vi "AutoBike FPGA backup.vi"() -> ()   [LabVIEW 2016]
doc: "The roboRIO FPGA Shipping Personality. This personality supports:\n- 8 Analog Input channels with 1 sample\n- 2 Analog Output channels with 1 sample\n- 30 Digital I/O channels with 1 sample\n- 1 RSL channel\n- 4 Relay channels\n- 1 Button\n- 3 LEDs\n- 1 Accelerometer\n- 13 PWM channels\n- 6 Encoder channels\n- 2 SPI channels\n- 2 I2C channels\n- 2 UART channels\n- 1 CAN channel\n- 2 Analog Input Interrupt\n- 5 Digital Input Interrupt\n- 1 Timer Interrupt"
uses:
  <vilib>/Platform/TimedLoop/XDataNode/wakeup.ctl
  <vilib>/Platform/TimedLoop/XDataNode/XDNodeRunTimeDep.lvlib
  <vilib>/Platform/TimedLoop/XDataNode/nitl_modes.ctl
  <vilib>/Platform/TimedLoop/XDataNode/timing_clust.ctl
  <vilib>/Platform/TimedLoop/XDataNode/XDataNode.xnode
  <vilib>/eio/EIONode/EIONode.xnode
  <vilib>/rvi/eio/common/nirviEmuTemplateMethod_errors.vi
  <vilib>/rvi/LocalResourceManager/LocalResourceManager.xnode
  <vilib>/rvi/DataTransferAndStorage/Container/Common/niFpgaContainerGetUniqueNameForEmu.vi
  <vilib>/rvi/DataTransferAndStorage/Container/Common/niFpgaContainerSetEmuInfo.vi
  <vilib>/rvi/eio/common/nirviEmuReportErrorAndStop.vi
  <vilib>/rvi/DataTransferAndStorage/Container/XNode/niFpgaContainer.xnode
  <vilib>/rvi/FIFO/Fifo_Resource/nirvififoEmulationRead.vi
  <vilib>/rvi/FIFO/Fifo_Resource/nirvififoEmulationWrite.vi
  Sub VIs/Utilities/Start Boolean.ctl
panel:
  out "DIO.SPI_CS3:0.IN":u8 format="%08b"
  in  "DIO.SPI_CS3:0.DIR":u8 format="%08b"
  in  "DIO.SPI_CS3:0.OUT":u8 format="%08b"
  in  "IRQ.TIMER.SETTIME":T1
  in  "IRQ.TIMER.WRITE":u32
  out "IRQ.TIMER.READ":u32
  in  "IRQ.DI_BTN.NO":u8
  in  "IRQ.DI_BTN.CNT":u32
  in  "IRQ.DI_BTN.FALL":bool
  in  "IRQ.DI_BTN.RISE":bool
  in  "IRQ.DI_BTN.ENA":bool
  in  "IRQ.AI_B_0.HYSTERESIS":u16=17
  in  "IRQ.AI_B_1.HYSTERESIS":u16=17
  in  "IRQ.AI_B_1.NO":u8
  in  "IRQ.AI_B_0.NO":u8
  in  "IRQ.AI_B_1.THRESHOLD":u16
  in  "IRQ.AI_B_0.THRESHOLD":u16
  in  "IRQ.AI_B_3:0.CNFG":u8 format="%.0b"
  in  "IRQ.DIO_B_0.NO":u8
  in  "IRQ.DIO_B_1.NO":u8
  in  "IRQ.DIO_B_2.NO":u8
  in  "IRQ.DIO_B_3.NO":u8
  in  "IRQ.DIO_B_3.CNT":u32
  in  "IRQ.DIO_B_2.CNT":u32
  in  "IRQ.DIO_B_1.CNT":u32
  in  "IRQ.DIO_B_0.CNT":u32
  in  "IRQ.DIO_B_7:0.FALL":u8 format="%08b"
  in  "IRQ.DIO_B_7:0.RISE":u8 format="%08b"
  in  "IRQ.DIO_B_7:0.ENA":u8 format="%08b"
  in  "SPI.SPI.IRQ.NO":u8=15
  in  "SPI.B.IRQ.NO":u8=15
  out "DIO.DIO_9:8.IN":u8 format="%08b"
  in  "ENC.DIO_3.CNFG":u8 format="%08b"
  out "ENC.DIO_3.CNTR":u32
  out "ENC.DIO_3.STAT":u8 format="%08b"
  in  "ENC.DIO_4.CNFG":u8 format="%08b"
  out "ENC.DIO_4.CNTR":u32
  out "ENC.DIO_4.STAT":u8 format="%08b"
  in  "DIO.DIO_9:8.OUT":u8 format="%08b"
  in  "DIO.DIO_9:8.DIR":u8 format="%08b"
  in  "ENC.DIO_2.CNFG":u8 format="%08b"
  out "ENC.DIO_2.CNTR":u32
  out "ENC.DIO_2.STAT":u8 format="%08b"
  out "ENC.DIO_1.STAT":u8 format="%08b"
  out "ENC.DIO_1.CNTR":u32
  in  "ENC.DIO_1.CNFG":u8 format="%08b"
  out "DIO.DIO_7:0.IN":u8 format="%08b"
  in  "SYS.SELECTDIO":u8 format="%08b"
  in  "DIO.DIO_7:0.DIR":u8 format="%08b"
  in  "DIO.DIO_7:0.OUT":u8 format="%08b"
  out "ENC.DIO_0.STAT":u8 format="%08b"
  out "ENC.DIO_0.CNTR":u32
  in  "ENC.DIO_0.CNFG":u8 format="%08b"
  out "DI.BTN":u8 format="%08b"
  in  "DO.LED 5:0":u8 format="%06b"
  in  "DO.RSL.OUT":bool
  out "SPI.SPI.STAT":u8 format="%08b"
  in  "SPI.SPI.GO":T1
  in  "SPI.SPI.CNT":u16
  in  "SPI.SPI.CNFG":u16 format="%016b"
  out "SPI.SPI.DATI":u16
  in  "SPI.SPI.DATO":u16
  out "I2C.I2C.DATI":u8
  out "I2C.I2C.STAT":u8 format="%08b"
  in  "I2C.I2C.DATO":u8
  in  "I2C.I2CADDR":u8 format="%08b"
  in  "I2C.I2C.CNTR":u8
  in  "I2C.I2C.CNTL":u8 format="%08b"
  in  "I2C.I2C.CNFG":u8 format="%08b"
  in  "I2C.I2C.GO":T1
  out "ACC.Z.VAL":u16
  out "ACC.Y.VAL":u16
  out "ACC.X.VAL":u16
  in  "DO.RELAY.OUT":u8 format="%08b"
  out "SYS.ACC.RDY":bool
  out "SYS.RDY":bool
  in  "PWM.PWM_5.MAX":u16
  in  "PWM.PWM_5.CMP":u16
  in  "PWM.PWM_5.CNFG":u8 format="%08b"
  in  "PWM.PWM_5.CS":u8
  out "PWM.PWM_5.CNTR":u16
  in  "PWM.PWM_6.MAX":u16
  in  "PWM.PWM_6.CMP":u16
  in  "PWM.PWM_6.CNFG":u8 format="%08b"
  in  "PWM.PWM_6.CS":u8
  out "PWM.PWM_6.CNTR":u16
  in  "PWM.PWM_7.MAX":u16
  in  "PWM.PWM_7.CMP":u16
  in  "PWM.PWM_7.CNFG":u8 format="%08b"
  in  "PWM.PWM_7.CS":u8
  out "PWM.PWM_7.CNTR":u16
  in  "PWM.PWM_8.MAX":u16
  in  "PWM.PWM_8.CMP":u16
  in  "PWM.PWM_8.CNFG":u8 format="%08b"
  in  "PWM.PWM_8.CS":u8
  out "PWM.PWM_8.CNTR":u16
  in  "PWM.PWM_9.MAX":u16
  in  "PWM.PWM_9.CMP":u16
  in  "PWM.PWM_9.CNFG":u8 format="%08b"
  in  "PWM.PWM_9.CS":u8
  out "PWM.PWM_9.CNTR":u16
  in  "PWM.PWM_4.MAX":u16
  in  "PWM.PWM_4.CMP":u16
  in  "PWM.PWM_4.CNFG":u8 format="%08b"
  in  "PWM.PWM_4.CS":u8
  out "PWM.PWM_4.CNTR":u16
  in  "PWM.PWM_3.MAX":u16
  in  "PWM.PWM_3.CMP":u16
  in  "PWM.PWM_3.CNFG":u8 format="%08b"
  in  "PWM.PWM_3.CS":u8
  out "PWM.PWM_3.CNTR":u16
  in  "PWM.PWM_2.MAX":u16
  in  "PWM.PWM_2.CMP":u16
  in  "PWM.PWM_2.CNFG":u8 format="%08b"
  in  "PWM.PWM_2.CS":u8
  out "PWM.PWM_2.CNTR":u16
  in  "PWM.PWM_1.MAX":u16
  in  "PWM.PWM_1.CMP":u16
  in  "PWM.PWM_1.CNFG":u8 format="%08b"
  in  "PWM.PWM_1.CS":u8
  out "PWM.PWM_1.CNTR":u16
  out "PWM.PWM_0.CNTR":u16
  in  "PWM.PWM_0.CS":u8
  in  "PWM.PWM_0.CNFG":u8 format="%08b"
  in  "PWM.PWM_0.CMP":u16
  in  "PWM.PWM_0.MAX":u16
  in  "AO.B_0.VAL":u16
  in  "AO.B_1.VAL":u16
  in  "AO.SYS.GO":T1
  out "AO.SYS.STAT":bool
  out "AI.B_0.VAL":u16
  out "AI.B_1.VAL":u16
  out "AI.B_2.VAL":u16
  out "AI.B_3.VAL":u16
  out "AI.AI_0.VAL":u16
  out "AI.AI_1.VAL":u16
  out "AI.AI_2.VAL":u16
  out "AI.AI_3.VAL":u16
  out "SYS.AI.RDY":bool
  in  "SYS.SELECTB":u8 format="%08b"
  in  "DIO.B_7:0.OUT":u8 format="%08b"
  in  "DIO.B_7:0.DIR":u8 format="%08b"
  out "DIO.B_7:0.IN":u8 format="%08b"
  in  "DIO.B_15:8.OUT":u8 format="%08b"
  in  "DIO.B_15:8.DIR":u8 format="%08b"
  out "DIO.B_15:8.IN":u8 format="%08b"
  in  "SPI.B.DATO":u16
  out "SPI.B.DATI":u16
  in  "SPI.B.CNFG":u16 format="%016b"
  in  "SPI.B.CNT":u16
  in  "SPI.B.GO":T1
  out "SPI.B.STAT":u8 format="%08b"
  in  "PWM.B_0.MAX":u16
  in  "PWM.B_0.CMP":u16
  in  "PWM.B_0.CNFG":u8 format="%08b"
  in  "PWM.B_0.CS":u8
  out "PWM.B_0.CNTR":u16
  in  "PWM.B_1.CMP":u16
  in  "PWM.B_1.MAX":u16
  out "PWM.B_1.CNTR":u16
  in  "PWM.B_1.CNFG":u8 format="%08b"
  in  "PWM.B_1.CS":u8
  in  "PWM.B_2.CMP":u16
  in  "PWM.B_2.MAX":u16
  out "PWM.B_2.CNTR":u16
  in  "PWM.B_2.CNFG":u8 format="%08b"
  in  "PWM.B_2.CS":u8
  in  "I2C.B.DATO":u8
  out "I2C.B.DATI":u8
  in  "I2C.B.ADDR":u8 format="%08b"
  in  "I2C.B.CNTR":u8
  in  "I2C.B.CNTL":u8 format="%08b"
  out "I2C.B.STAT":u8 format="%08b"
  in  "I2C.B.CNFG":u8 format="%08b"
  in  "I2C.B.GO":T1
  in  "ENC.B.CNFG":u8 format="%08b"
  out "ENC.B.CNTR":u32
  out "ENC.B.STAT":u8 format="%08b"
  # "System"
  # "Onboard Devices"
  # "Connector B"
  # "DIO"
  # "SPI"
  # "PWM"
  # "I2C"
  # "AI"
  # "RELAY"
  # "RSL"
  # "Accelerometer"
  # "SPI Master"
  # "Analog Input"
  # "Analog Output"
  # "Digital I/O"
  # "Counters / PWM"
  # "Digital I/O"
  # "Encoders"
  # "IO Configuration"
  # "Buttons & LEDs"
  # "SPI CS DIO"
  # "Analog Interrupt"
  # "Digital Interrupt"
  # "Encoders"
  # "IO Configuration"
  # "Button Interrupt"
  # "I2C Master"
  # "FPGA Timer"
  # "This VI contains the default FPGA personality in addition to code that generates a sine waveform and filtered sine waveform based on parameters set by RT Main.vi. Keeping the default personality allows you to continue using the roboRIO APIs even after adding custom FPGA code."
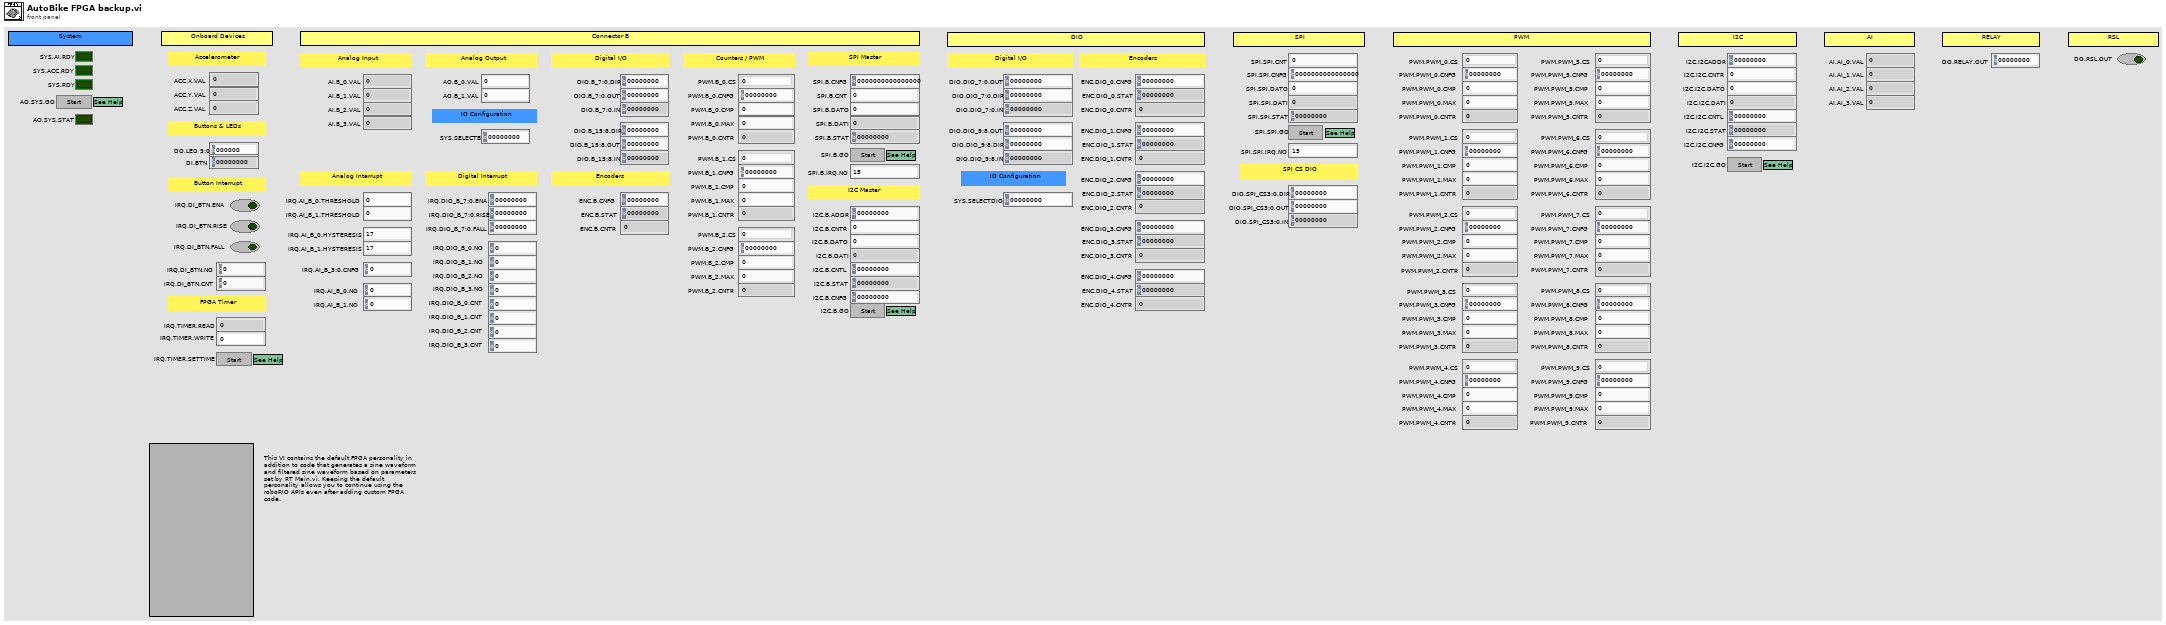
[diagram p1: front panel]
types:
  T1 = typedef "Start Boolean.ctl" = bool
  T2 = typedef "XDNodeRunTimeDep.lvlib/timing_clust.ctl" = cluster{"Expected End [f-1]":u64, "Actual End [f-1]":u64, "Finished Late? [f-1]":bool, "Expected End [i-1]":u64, "Actual End [i-1]":u64, "Finished Late? [i-1]":bool, "Expected Start [i]":u64, "Actual Start [i]":u64, "Expected Start [f]":u64, "Actual Start [f]":u64, "Source Name":string, "Structure Name":string, "Period":i64, "Deadline":i64, "Offset":i64, "Start":i64, "Priority":i32, "Timeout":i32, "Mode":T3, "Wakeup Reason":T4, "Error":errorcluster, "Source Type":string, "Secondary Source Type":string, "Global End Time":u64, "Global Start Time":u64, "Frame Duration":u64, "Iteration Duration":u64, "Assigned CPU":i32, "I/O Scan Engine Mode":u32}
  T3 = typedef "XDNodeRunTimeDep.lvlib/nitl_modes.ctl" = enum32{"No Change", "Process missed periods, maintain original phase", "Discard missed periods, maintain original phase", "Process missed periods, ignore original phase", "Discard missed periods, ignore original phase"}
  T4 = typedef "XDNodeRunTimeDep.lvlib/wakeup.ctl" = enum32{"Normal", "Aborted", "Asynchronous wakeup", "Timing source error", "Timed loop error", "Timeout"}
diagram:
  # "The accelerometer nodes take some time before the FPGA can first read the values. This is because it takes time to read from the accelerometer. An iteration of the While Loop will not complete until the accelerometer values have been read.\n\nAfter the completion of the first iteration of the While Loop, all indicators have valid values."
  # "The analog output nodes take some time before the FPGA write the values to the pins. The GO and STAT registers are used to handshake between the FPGA and host. When the host wants the values to be written, the host sets the GO register to TRUE. If the host reads the STAT register before setting the value of the GO register, it can wait for the value of the STAT register to invert. The value inversion tells the host that the output values have been written."
  # "The FPGA timer fires the interrupt request (IRQ) when TIMER.Read counts down to zero. If TIMER.Read is not zero, it counts down to one per microsecond."
  # "The analog input nodes take some time before the FPGA can first read the values. This is because it takes time to set up the Analog-to-Digital converter (ADC) and convert the first reading. An iteration of the While Loop will not complete until all the analog input channels have been sampled.\n\nAfter the completion of the first iteration of the While Loop, all indicators have valid values."
  # "Note: On some hardware a \"ghosting effect\" may occur on any unconnected AI channels. For example, if channel AI0 is connected and channels AI1~AI7 are not connected the the value read at AI0 may be seen on indicators AI1~AI7. This is common for hardware that use a multiplexed (MUXed) Analog-to-Digital converter (ADC), because the input analog signal is used to charge a capacitor which does not discharge before the unconnected channel is read.\n\nYou can hide the \"ghosting effect\" by using an mask register. This register is used to decide when the indicator should be updated."
  # "The only interface that sends interrupts to the RT side. Timer interrupts, analog input interrupts, digital input interrupts, and SPI interrupt share this interface.\n\nAll interrupts work in sequence. One interrupt waits until the previous interrupt request (IRQ) gets acknowledged on the RT side."
  # "NOTE: The SYS.RDY boolean MUST exist and must become TRUE at some point otherwise the myRIO API will not function correctly."
  # "There is some delay between when the FPGA code starts and the analog inputs, accelerometer, and scaling values outputs are valid. If the host wants to ensure that there are valid values in theses registers it should wait for each subsystem to finish its initialization process. \n\nWhen all subsystems have finished initializinig, the SYS.RDY indicator will be true, which can be polled by the host to determine the status of the FPGA. Alternatively, the host can poll the individual SYS.xx.RDY indicators to determine the status of the individual subsystems.\n\nThis loop continues indefinitely, essentially making SYS.RDY a read-only register."
  n1 = while {
    stop <- FALSE stop-if-true
    # "Host Synchronization"
    n2 = local read "SYS.ACC.RDY"() -> (w23:bool)
    n3 = local read "SYS.AI.RDY"() -> (w25:bool)
    n4 = Compound Arithmetic op=AND(w25, w23) -> (→"SYS.RDY":bool)
  }
  n5 = while {
    stop <- FALSE stop-if-true
    # "Interrupt to RT"
    n6 = xnode ("FIFO Method Node")("Timeout"=-1) -> ("Element"=w28:u8)  [unwired: 1 in, 2 out]
    n7 = call <vilib>:"niFPGA Interrupt.vi"("Wait Until Cleared (F)"=TRUE, "IRQ Number (0)"=w28) -> ()  [unwired: 1 in]
  }
  n8 = while {
    stop <- FALSE stop-if-true
    # "Timer"
    n9 = local read "IRQ.TIMER.READ"() -> (w33:u32)
    n10 = Select(t="IRQ.TIMER.WRITE", s="IRQ.TIMER.SETTIME", f=w33) -> (s? t:f=w31:u32)
    n11 = case shown="Default" w31 {
      selector: w31 -> [w37 w40]
      tunnel: [w37 w38] -> w30
      frame 0 {
      }
      frame Default {
        n12 = Decrement(x=w40) -> (x-1=w39:u32)
        n13 = case shown="0" w39 {
          selector: w39 -> [w41 w44]
          tunnel: [w41 w44] -> w38
          frame Default {
          }
          frame 0 {
            w43 = u8 0  # Reserved for Timer IRQ
            n14 = xnode ("FIFO Method Node")("Element"=w43, "Timeout"=-1) -> ()  [unwired: 1 in, 2 out]
          }
        }
      }
    }
    "IRQ.TIMER.READ" <- w30
    n15 = call "Loop Timer"("Count(uSec)"=u8 1 ("Count(mSec)")) -> ()  [unwired: 1 out]
  }
  n16 = xnode "VI-Defined FIFO Configuration"() -> ("FIFO Out"=w2:refnum<k21>)
  n17 = while {
    tunnel: w2 -> [w53]
    i -> [w67]
    stop <- FALSE stop-if-true
    # "Analog Input"
    n18 = Greater Than 0?(x=w67) -> (x > 0?=→"SYS.AI.RDY":bool)
    n19 = xnode "FPGA I/O Node"() -> ("MXP/AI0"=w46, "MXP/AI1"=w45, "MXP/AI2"=→"AI.B_2.VAL", "MXP/AI3"=→"AI.B_3.VAL", "AnalogIn0"=→"AI.AI_0.VAL", "AnalogIn1"=→"AI.AI_1.VAL", "AnalogIn2"=→"AI.AI_2.VAL", "AnalogIn3"=→"AI.AI_3.VAL")  [unwired: 8 in, 8 out]
    "AI.B_0.VAL" <- w46
    "AI.B_1.VAL" <- w45
    n20 = Number To Boolean Array(number="IRQ.AI_B_3:0.CNFG") -> (Boolean array=w54:bool[])
    n21 = Index Array(array=w54) -> (element #1=w56:bool, element #2=w57:bool, element #3=w59:bool, element #4=w60:bool)  [unwired: 4 in]
    n22 = call "Check AI IRQ.vi"("Hysteresis"="IRQ.AI_B_1.HYSTERESIS", "FIFO In"=w53, "IRQ Number"="IRQ.AI_B_1.NO", "Threshold"="IRQ.AI_B_1.THRESHOLD", "Analog Value"=w45, "Rising Edge?"=w60, "Enable Interrupt?"=w59) -> ()  [unwired: 5 in]
    n23 = call "Check AI IRQ.vi"("Hysteresis"="IRQ.AI_B_0.HYSTERESIS", "FIFO In"=w53, "IRQ Number"="IRQ.AI_B_0.NO", "Threshold"="IRQ.AI_B_0.THRESHOLD", "Analog Value"=w46, "Rising Edge?"=w57, "Enable Interrupt?"=w56) -> ()  [unwired: 5 in]
  }
  n24 = while {
    stop <- FALSE stop-if-true
    # "Analog Output"
    n25 = feedback #1(FALSE) -> (w71:bool)
    n26 = case shown="True" "AO.SYS.GO" {
      tunnel: "AO.B_0.VAL" -> [_ w81]
      tunnel: "AO.B_1.VAL" -> [_ w80]
      tunnel: w71 -> [w76 w79]
      tunnel: [w76 w77] -> w69
      frame False {
      }
      frame True {
        n27 = flat-sequence {
          tunnel: w81 -> [w84]
          tunnel: w80 -> [w83]
          tunnel: w79 -> [w82]
          tunnel: [w82] -> w78
          tunnel: w78 -> [w86]
          tunnel: [w85] -> w77
          frame #0 {
            n28 = xnode "FPGA I/O Node"("MXP/AO0"=w84, "MXP/AO1"=w83) -> ()  [unwired: 2 in, 2 out]
          }
          frame #1 {
            n29 = Not(x=w86) -> (.not. x?=w85:bool)
          }
        }
      }
    }
    "AO.SYS.STAT" <- w69
    n30 = feedback-in #1(w69) -> ()
  }
  n31 = while {
    i -> [w94]
    stop <- FALSE stop-if-true
    # "Onboard Accelerometer"
    n32 = xnode "FPGA I/O Node"() -> ("AccelerationX"=w92, "AccelerationY"=w91, "AccelerationZ"=w90)  [unwired: 3 in, 3 out]
    n33 = Greater Than 0?(x=w94) -> (x > 0?=→"SYS.ACC.RDY":bool)
    n34 = To Unsigned Word Integer(number=w92) -> (unsigned 16bit integer=→"ACC.X.VAL":u16)
    n35 = To Unsigned Word Integer(number=w91) -> (unsigned 16bit integer=→"ACC.Y.VAL":u16)
    n36 = To Unsigned Word Integer(number=w90) -> (unsigned 16bit integer=→"ACC.Z.VAL":u16)
  }
  n37 = xnode "VI-Defined FIFO Configuration"() -> ("FIFO Out"=w1:refnum<k21>)
  n38 = node-c288() -> (w7:T2)  [unwired: 1 in]
  n39 = timed-loop {
    timing: w7 -> [_]
    timing-out: [_] -> w6
    tunnel: w1 -> [w101]
    stop <- FALSE stop-if-true
    # "Button IRQ"
    # "Onboard DIO"
    n40 = xnode "FPGA I/O Node"() -> ("User Button"=w102)  [unwired: 1 in, 1 out]
    n41 = Number To Boolean Array(number="DO.LED 5:0") -> (Boolean array=w112:bool[])
    n42 = Index Array(array=w112) -> (element #1=w110:bool, element #2=w109:bool, element #3=w108:bool, element #4=w107:bool, element #5=w106:bool, element #6=w105:bool)  [unwired: 6 in]
    n43 = Build Array(w102) -> (w104:void[])
    n44 = call "DIO IRQ 1-bit.vi"("IRQ.NO"="IRQ.DI_BTN.NO", "IRQ.CNT"="IRQ.DI_BTN.CNT", "FIFO in"=w101, "IRQ.FALL"="IRQ.DI_BTN.FALL", "IRQ.RISE"="IRQ.DI_BTN.RISE", "IRQ.ENA"="IRQ.DI_BTN.ENA", "DIO"=w102) -> ()  [unwired: 5 in]
    n45 = Boolean Array To Number(Boolean array=w104) -> (number=→"DI.BTN":u8)
    n46 = xnode "FPGA I/O Node"("Radio LED Green"=w110, "Radio LED Red"=w109, "Comm LED Green"=w108, "Comm LED Red"=w107, "Mode LED Green"=w106, "Mode LED Red"=w105) -> ()  [unwired: 6 in, 6 out]
  }
  n47 = while {
    stop <- FALSE stop-if-true
    # "Button SCTL Interrupt Buffer"
    n48 = feedback #2(u8 0 ("Element")) -> (w118:u8)
    n49 = feedback #3(FALSE ("Timed Out?")) -> (w122:bool)
    n50 = case shown="False" w122 {
      tunnel: [w124 w126] -> w119
      tunnel: w118 -> [_ w126]
      frame False {
        n51 = xnode ("FIFO Read")("Timeout"=-1) -> ("Element"=w124:u8)  [unwired: 1 in, 2 out]
      }
      frame True {
      }
    }
    n52 = feedback-in #2(w119) -> ()
    n53 = xnode ("FIFO Method Node")("Element"=w119, "Timeout"=0) -> ("Timed Out?"=w120:bool)  [unwired: 1 in, 1 out]
    n54 = feedback-in #3(w120) -> ()
  }
  n55 = node-c288(w6) -> ()
  n56 = xnode "VI-Defined FIFO Configuration"() -> ("FIFO Out"=w5:refnum<k21>)
  n57 = xnode "VI-Defined FIFO Configuration"() -> ("FIFO Out"=w3:refnum<k21>)
  n58 = node-c288() -> (w21:T2)  [unwired: 1 in]
  n59 = timed-loop {
    timing: w21 -> [_]
    timing-out: [_] -> w20
    tunnel: w5 -> [w163]
    tunnel: w3 -> [w151]
    stop <- _ stop-if-true
    # "DIO/ IRQ"
    # "DIO / Encoder"
    # "DIO / I2C Master"
    # "DIO / PWM"
    # "DIO"
    # "DIO"
    # "DIO/ SPI Master"
    # "Connector MXP DIO"
    n60 = call "Split HDC Bank1 DIO.vi"("IN 7:0"="DIO.B_7:0.OUT") -> ("OUT 3:0"=w251:fxp<+,4,4>, "OUT 4"=w166:bool, "OUT 7:5"=w248:fxp<+,3,3>)
    n61 = call "Split HDC Bank1 DIO.vi"("IN 7:0"="DIO.B_7:0.DIR") -> ("OUT 3:0"=w250:fxp<+,4,4>, "OUT 4"=w249:bool, "OUT 7:5"=w247:fxp<+,3,3>)
    n62 = call "Split HDC Function Select.vi"("IN 7:0"="SYS.SELECTB") -> ("OUT 1:0"=w187:fxp<+,2,2>, "OUT 7"=w182:bool, "OUT 2"=w186:bool, "OUT 3"=w185:bool, "OUT 4"=w184:bool, "OUT 5"=w183:bool)
    n63 = call "DIO 4-bit.vi"("DIO0 Refnum"=refnum<k21> "MXP/DIO0", "DIO1 Refnum"=refnum<k21> "MXP/DIO1", "DIO2 Refnum"=refnum<k21> "MXP/DIO2", "DIR 3:0"=w250, "OUT 3:0"=w251, "DIO3 Refnum"=refnum<k21> "MXP/DIO3") -> ("IN 3:0"=w162:fxp<+,4,4>)  [unwired: 5 in]
    n64 = call "DIO 1-bit.vi"("DIR"=w249, "OUT"=w166, "DIO Refnum"=refnum<k21> "MXP/DIO4") -> ("IN"=w223:bool)  [unwired: 8 in]
    n65 = call "DIO_SPI.vi"("DIO.2:0.OUT"=w248, "DIO.2:0.DIR"=w247, "SPI.CNT"="SPI.B.CNT", "SPI.CNFG"="SPI.B.CNFG", "SPI.DATO"="SPI.B.DATO", "SPI.GO"="SPI.B.GO", "DIO.2/SPI.MOSI Refnum"=refnum<k21> "MXP/DIO7" ("DIO.2/SPI.SCLK"), "SELECT.1:0"=w187, "DIO.1/SPI.MISO Refnum"=refnum<k21> "MXP/DIO6" ("DIO.1/SPI.MOSI"), "DIO.0/SPI.SCLK Refnum"=refnum<k21> "MXP/DIO5" ("DIO.0/SPI.MISO")) -> ("DIO.2:0.IN"=w222:fxp<+,3,3>, "SPI.DATI"=→"SPI.B.DATI":u16, "SPI.STAT"=w165:u8)  [unwired: 7 in]
    "SPI.B.STAT" <- w165
    n66 = call "SPI IRQ.vi"("SPI.A.IRQ.NO"="SPI.B.IRQ.NO", "SPI.STAT"=w165, "FIFO In"=w163) -> ()  [unwired: 9 in]
    n67 = call "Join HDC Bank1 DIO.vi"("IN 7:5"=w222, "IN 4"=w223, "IN 3:0"=w162) -> ("OUT 7:0"=→"DIO.B_7:0.IN":u8)
    n68 = Number To Boolean Array(number="IRQ.DIO_B_7:0.ENA") -> (Boolean array=w148:bool[])
    n69 = Number To Boolean Array(number="IRQ.DIO_B_7:0.RISE") -> (Boolean array=w139:bool[])
    n70 = Number To Boolean Array(number="IRQ.DIO_B_7:0.FALL") -> (Boolean array=w134:bool[])
    n71 = Index Array(array=w148) -> (element #1=w149:bool, element #2=w147:bool, element #3=w146:bool, element #4=w145:bool)  [unwired: 4 in]
    n72 = Index Array(array=w139) -> (element #1=w138:bool, element #2=w140:bool, element #3=w141:bool, element #4=w142:bool)  [unwired: 4 in]
    n73 = Index Array(array=w134) -> (element #1=w135:bool, element #2=w133:bool, element #3=w132:bool, element #4=w131:bool)  [unwired: 4 in]
    n74 = Build Array(w149, w147, w146, w145) -> (w150:bool[])
    n75 = Build Array(w138, w140, w141, w142) -> (w137:bool[])
    n76 = Build Array(w135, w133, w132, w131) -> (w136:bool[])
    n77 = Build Array("IRQ.DIO_B_0.CNT", "IRQ.DIO_B_1.CNT", "IRQ.DIO_B_2.CNT", "IRQ.DIO_B_3.CNT") -> (w157:u32[])
    n78 = Build Array("IRQ.DIO_B_0.NO", "IRQ.DIO_B_1.NO", "IRQ.DIO_B_2.NO", "IRQ.DIO_B_3.NO") -> (w152:u8[])
    n79 = Boolean Array To Number(Boolean array=w150) -> (number=w143:fxp<+,4,4>)
    n80 = Boolean Array To Number(Boolean array=w137) -> (number=w128:fxp<+,4,4>)
    n81 = Boolean Array To Number(Boolean array=w136) -> (number=w127:fxp<+,4,4>)
    n82 = call "DIO IRQ 4-bit.vi"("IRQ NO"=w152, "IRQ CNT"=w157, "FIFO In"=w151, "IRQ.FALL"=w127, "IRQ.RISE"=w128, "IRQ.ENA"=w143, "IN 3:0"=w162) -> ()  [unwired: 5 in]
    n83 = call "Split HDC Bank2 DIO.vi"("IN 7:0"="DIO.B_15:8.OUT") -> ("OUT 5"=w168:bool, "OUT 7:6"=w192:fxp<+,2,2>, "OUT 4:3"=w170:fxp<+,2,2>, "OUT 2"=w172:bool, "OUT 0"=w176:bool, "OUT 1"=w175:bool)  [unwired: 2 in]
    n84 = call "Split HDC Bank2 DIO.vi"("IN 7:0"="DIO.B_15:8.DIR") -> ("OUT 5"=w167:bool, "OUT 7:6"=w191:fxp<+,2,2>, "OUT 4:3"=w169:fxp<+,2,2>, "OUT 2"=w171:bool, "OUT 0"=w174:bool, "OUT 1"=w173:bool)  [unwired: 2 in]
    n85 = call "DIO_PWM.vi"("DIO.OUT"=w176, "DIO.DIR"=w174, "PWM.CS"="PWM.B_0.CS", "PWM.CNFG"="PWM.B_0.CNFG", "PWM.CMP"="PWM.B_0.CMP", "PWM.MAX"="PWM.B_0.MAX", "DIO/PWM"=refnum<k21> "MXP/DIO8", "SELECT"=w186) -> ("DIO.IN"=w181:bool, "PWM.CNTR"=→"PWM.B_0.CNTR":u16)  [unwired: 10 in]
    n86 = call "DIO_PWM.vi"("DIO.OUT"=w175, "DIO.DIR"=w173, "PWM.CS"="PWM.B_1.CS", "PWM.CNFG"="PWM.B_1.CNFG", "PWM.CMP"="PWM.B_1.CMP", "PWM.MAX"="PWM.B_1.MAX", "DIO/PWM"=refnum<k21> "MXP/DIO9", "SELECT"=w185) -> ("DIO.IN"=w180:bool, "PWM.CNTR"=→"PWM.B_1.CNTR":u16)  [unwired: 10 in]
    n87 = call "DIO_PWM.vi"("DIO.OUT"=w172, "DIO.DIR"=w171, "PWM.CS"="PWM.B_2.CS", "PWM.CNFG"="PWM.B_2.CNFG", "PWM.CMP"="PWM.B_2.CMP", "PWM.MAX"="PWM.B_2.MAX", "DIO/PWM"=refnum<k21> "MXP/DIO10", "SELECT"=w184) -> ("DIO.IN"=w179:bool, "PWM.CNTR"=→"PWM.B_2.CNTR":u16)  [unwired: 10 in]
    n88 = call "DIO_Encoder.vi"("DIO.1:0.OUT"=w170, "DIO.1:0.DIR"=w169, "QE.CNFG"="ENC.B.CNFG", "DIO.1/QE.B"=refnum<k21> "MXP/DIO12", "SELECT"=w183, "DIO.0/QE.A"=refnum<k21> "MXP/DIO11") -> ("DIO.1:0.IN"=w178:fxp<+,2,2>, "QE.CNTR"=→"ENC.B.CNTR":u32, "QE.STAT"=→"ENC.B.STAT":u8)  [unwired: 11 in]
    n89 = call "DIO 1-bit.vi"("DIR"=w167, "OUT"=w168, "DIO Refnum"=refnum<k21> "MXP/DIO13") -> ("IN"=w177:bool)  [unwired: 8 in]
    n90 = call "DIO_I2C.vi"("DIO.1:0.OUT"=w192, "DIO.1:0.DIR"=w191, "I2C.CNFG"="I2C.B.CNFG", "I2C.CNTL"="I2C.B.CNTL", "I2C.ADDR"="I2C.B.ADDR", "I2C.DATO"="I2C.B.DATO", "DIO.1/I2C.SDA"=refnum<k21> "MXP/DIO15" ("DIO.1/I2C.SCL"), "I2C.CNTR"="I2C.B.CNTR", "DIO.0/I2C.SCL"=refnum<k21> "MXP/DIO14" ("DIO.0/I2C.SDA"), "Execute?"="I2C.B.GO", "SELECT"=w182) -> ("DIO.1:0.IN"=w189:fxp<+,2,2>, "I2C.DATI"=→"I2C.B.DATI":u8, "I2C.STAT"=→"I2C.B.STAT":u8)  [unwired: 6 in]
    n91 = call "Join HDC Bank2 DIO.vi"("IN 7:6"=w189, "IN 5"=w177, "IN 4:3"=w178, "IN 0"=w181, "IN 2"=w179, "IN 1"=w180) -> ("OUT 7:0"=→"DIO.B_15:8.IN":u8)  [unwired: 4 in]
  }
  n92 = while {
    stop <- FALSE stop-if-true
    # "Connector A SPI SCTL Interrupt Buffer"
    n93 = feedback #4(u8 0 ("Element")) -> (w256:u8)
    n94 = feedback #5(FALSE ("Timed Out?")) -> (w260:bool)
    n95 = case shown="False" w260 {
      tunnel: [w262 w264] -> w257
      tunnel: w256 -> [_ w264]
      frame False {
        n96 = xnode ("FIFO Method Node")("Timeout"=-1) -> ("Element"=w262:u8)  [unwired: 1 in, 2 out]
      }
      frame True {
      }
    }
    n97 = feedback-in #4(w257) -> ()
    n98 = xnode ("FIFO Method Node")("Element"=w257, "Timeout"=0) -> ("Timed Out?"=w258:bool)  [unwired: 1 in, 1 out]
    n99 = feedback-in #5(w258) -> ()
  }
  n100 = while {
    stop <- FALSE stop-if-true
    # "Connector A DIO SCTL Interrupt Buffer"
    n101 = feedback #6(u8 0 ("Element")) -> (w267:u8)
    n102 = feedback #7(FALSE ("Timed Out?")) -> (w271:bool)
    n103 = case shown="False" w271 {
      tunnel: [w273 w275] -> w268
      tunnel: w267 -> [_ w275]
      frame False {
        n104 = xnode ("FIFO Method Node")("Timeout"=-1) -> ("Element"=w273:u8)  [unwired: 1 in, 2 out]
      }
      frame True {
      }
    }
    n105 = feedback-in #6(w268) -> ()
    n106 = xnode ("FIFO Method Node")("Element"=w268, "Timeout"=0) -> ("Timed Out?"=w269:bool)  [unwired: 1 in, 1 out]
    n107 = feedback-in #7(w269) -> ()
  }
  n108 = node-c288(w20) -> ()
  n109 = node-c288() -> (w15:T2)  [unwired: 1 in]
  n110 = timed-loop {
    timing: w15 -> [_]
    timing-out: [_] -> w14
    stop <- FALSE stop-if-true
    # "DIO"
    n111 = call "Split HDC Bank3 DIO.vi"("IN 7:0"="DIO.DIO_7:0.OUT") -> ("OUT 1:0"=w291:fxp<+,2,2>, "OUT 3:2"=w290:fxp<+,2,2>, "OUT 5:4"=w289:fxp<+,2,2>, "OUT 7:6"=w281:fxp<+,2,2>)
    n112 = call "Split HDC Bank3 DIO.vi"("IN 7:0"="DIO.DIO_7:0.DIR") -> ("OUT 1:0"=w287:fxp<+,2,2>, "OUT 3:2"=w286:fxp<+,2,2>, "OUT 5:4"=w285:fxp<+,2,2>, "OUT 7:6"=w280:fxp<+,2,2>)
    n113 = Number To Boolean Array(number="SYS.SELECTDIO") -> (Boolean array=w322:bool[])
    n114 = Index Array(array=w322) -> (element #1=w321:bool, element #2=w318:bool, element #3=w309:bool, element #4=w298:bool, element #5=w297:bool)  [unwired: 5 in]
    n115 = call "DIO_Encoder.vi"("DIO.1:0.OUT"=w281, "DIO.1:0.DIR"=w280, "QE.CNFG"="ENC.DIO_3.CNFG", "DIO.1/QE.B"=refnum<k21> "DIO/DIO7" ("DIO Refnum"), "SELECT"=w298, "DIO.0/QE.A"=refnum<k21> "DIO/DIO6" ("DIO Refnum")) -> ("DIO.1:0.IN"=w279:fxp<+,2,2>, "QE.CNTR"=→"ENC.DIO_3.CNTR":u32, "QE.STAT"=→"ENC.DIO_3.STAT":u8)  [unwired: 11 in]
    n116 = call "DIO_Encoder.vi"("DIO.1:0.OUT"=w291, "DIO.1:0.DIR"=w287, "QE.CNFG"="ENC.DIO_0.CNFG", "DIO.1/QE.B"=refnum<k21> "DIO/DIO1" ("DIO Refnum"), "SELECT"=w321, "DIO.0/QE.A"=refnum<k21> "DIO/DIO0" ("DIO Refnum")) -> ("DIO.1:0.IN"=w296:fxp<+,2,2>, "QE.CNTR"=→"ENC.DIO_0.CNTR":u32, "QE.STAT"=→"ENC.DIO_0.STAT":u8)  [unwired: 11 in]
    n117 = call "DIO_Encoder.vi"("DIO.1:0.OUT"=w290, "DIO.1:0.DIR"=w286, "QE.CNFG"="ENC.DIO_1.CNFG", "DIO.1/QE.B"=refnum<k21> "DIO/DIO3" ("DIO Refnum"), "SELECT"=w318, "DIO.0/QE.A"=refnum<k21> "DIO/DIO2" ("DIO Refnum")) -> ("DIO.1:0.IN"=w295:fxp<+,2,2>, "QE.CNTR"=→"ENC.DIO_1.CNTR":u32, "QE.STAT"=→"ENC.DIO_1.STAT":u8)  [unwired: 11 in]
    n118 = call "DIO_Encoder.vi"("DIO.1:0.OUT"=w289, "DIO.1:0.DIR"=w285, "QE.CNFG"="ENC.DIO_2.CNFG", "DIO.1/QE.B"=refnum<k21> "DIO/DIO5" ("DIO Refnum"), "SELECT"=w309, "DIO.0/QE.A"=refnum<k21> "DIO/DIO4" ("DIO Refnum")) -> ("DIO.1:0.IN"=w294:fxp<+,2,2>, "QE.CNTR"=→"ENC.DIO_2.CNTR":u32, "QE.STAT"=→"ENC.DIO_2.STAT":u8)  [unwired: 11 in]
    n119 = call "Join HDC Bank3 DIO.vi"("IN 7:6"=w279, "IN 5:4"=w294, "IN 3:2"=w295, "IN 1:0"=w296) -> ("OUT 7:0"=→"DIO.DIO_7:0.IN":u8)
    n120 = call "Split HDC Bank3 DIO.vi"("IN 7:0"="DIO.DIO_9:8.OUT") -> ("OUT 1:0"=w278:fxp<+,2,2>)  [unwired: 3 out]
    n121 = call "Split HDC Bank3 DIO.vi"("IN 7:0"="DIO.DIO_9:8.DIR") -> ("OUT 1:0"=w277:fxp<+,2,2>)  [unwired: 3 out]
    n122 = call "DIO_Encoder.vi"("DIO.1:0.OUT"=w278, "DIO.1:0.DIR"=w277, "QE.CNFG"="ENC.DIO_4.CNFG", "DIO.1/QE.B"=refnum<k21> "DIO/DIO9" ("DIO Refnum"), "SELECT"=w297, "DIO.0/QE.A"=refnum<k21> "DIO/DIO8" ("DIO Refnum")) -> ("DIO.1:0.IN"=w276:fxp<+,2,2>, "QE.CNTR"=→"ENC.DIO_4.CNTR":u32, "QE.STAT"=→"ENC.DIO_4.STAT":u8)  [unwired: 11 in]
    n123 = call "Join HDC Bank3 DIO.vi"("IN 1:0"=w276) -> ("OUT 7:0"=→"DIO.DIO_9:8.IN":u8)  [unwired: 3 in]
  }
  n124 = node-c288(w14) -> ()
  n125 = node-c288() -> (w19:T2)  [unwired: 1 in]
  n126 = timed-loop {
    timing: w19 -> [_]
    timing-out: [_] -> w18
    stop <- FALSE stop-if-true
    # "PWM"
    n127 = call "PWM (Single Output).vi"("Clock Select"="PWM.PWM_0.CS", "Counter Control"="PWM.PWM_0.CNFG", "Output Compare Value"="PWM.PWM_0.CMP", "Max Counter Value"="PWM.PWM_0.MAX") -> ("Output"=w387:bool, "Counter Value"=→"PWM.PWM_0.CNTR":u16)  [unwired: 6 in]
    n128 = call "PWM (Single Output).vi"("Clock Select"="PWM.PWM_1.CS", "Counter Control"="PWM.PWM_1.CNFG", "Output Compare Value"="PWM.PWM_1.CMP", "Max Counter Value"="PWM.PWM_1.MAX") -> ("Output"=w381:bool, "Counter Value"=→"PWM.PWM_1.CNTR":u16)  [unwired: 6 in]
    n129 = call "PWM (Single Output).vi"("Clock Select"="PWM.PWM_2.CS", "Counter Control"="PWM.PWM_2.CNFG", "Output Compare Value"="PWM.PWM_2.CMP", "Max Counter Value"="PWM.PWM_2.MAX") -> ("Output"=w365:bool, "Counter Value"=→"PWM.PWM_2.CNTR":u16)  [unwired: 6 in]
    n130 = call "PWM (Single Output).vi"("Clock Select"="PWM.PWM_3.CS", "Counter Control"="PWM.PWM_3.CNFG", "Output Compare Value"="PWM.PWM_3.CMP", "Max Counter Value"="PWM.PWM_3.MAX") -> ("Output"=w364:bool, "Counter Value"=→"PWM.PWM_3.CNTR":u16)  [unwired: 6 in]
    n131 = call "PWM (Single Output).vi"("Clock Select"="PWM.PWM_4.CS", "Counter Control"="PWM.PWM_4.CNFG", "Output Compare Value"="PWM.PWM_4.CMP", "Max Counter Value"="PWM.PWM_4.MAX") -> ("Output"=w363:bool, "Counter Value"=→"PWM.PWM_4.CNTR":u16)  [unwired: 6 in]
    n132 = xnode "FPGA I/O Node"("PWM/PWM0"=w387, "PWM/PWM1"=w381, "PWM/PWM2"=w365, "PWM/PWM3"=w364, "PWM/PWM4"=w363) -> ()  [unwired: 5 in, 5 out]
    n133 = call "PWM (Single Output).vi"("Clock Select"="PWM.PWM_5.CS", "Counter Control"="PWM.PWM_5.CNFG", "Output Compare Value"="PWM.PWM_5.CMP", "Max Counter Value"="PWM.PWM_5.MAX") -> ("Output"=w338:bool, "Counter Value"=→"PWM.PWM_5.CNTR":u16)  [unwired: 6 in]
    n134 = call "PWM (Single Output).vi"("Clock Select"="PWM.PWM_6.CS", "Counter Control"="PWM.PWM_6.CNFG", "Output Compare Value"="PWM.PWM_6.CMP", "Max Counter Value"="PWM.PWM_6.MAX") -> ("Output"=w344:bool, "Counter Value"=→"PWM.PWM_6.CNTR":u16)  [unwired: 6 in]
    n135 = call "PWM (Single Output).vi"("Clock Select"="PWM.PWM_7.CS", "Counter Control"="PWM.PWM_7.CNFG", "Output Compare Value"="PWM.PWM_7.CMP", "Max Counter Value"="PWM.PWM_7.MAX") -> ("Output"=w360:bool, "Counter Value"=→"PWM.PWM_7.CNTR":u16)  [unwired: 6 in]
    n136 = call "PWM (Single Output).vi"("Clock Select"="PWM.PWM_8.CS", "Counter Control"="PWM.PWM_8.CNFG", "Output Compare Value"="PWM.PWM_8.CMP", "Max Counter Value"="PWM.PWM_8.MAX") -> ("Output"=w361:bool, "Counter Value"=→"PWM.PWM_8.CNTR":u16)  [unwired: 6 in]
    n137 = call "PWM (Single Output).vi"("Clock Select"="PWM.PWM_9.CS", "Counter Control"="PWM.PWM_9.CNFG", "Output Compare Value"="PWM.PWM_9.CMP", "Max Counter Value"="PWM.PWM_9.MAX") -> ("Output"=w362:bool, "Counter Value"=→"PWM.PWM_9.CNTR":u16)  [unwired: 6 in]
    n138 = xnode "FPGA I/O Node"("PWM/PWM5"=w338, "PWM/PWM6"=w344, "PWM/PWM7"=w360, "PWM/PWM8"=w361, "PWM/PWM9"=w362) -> ()  [unwired: 5 in, 5 out]
  }
  n139 = node-c288(w18) -> ()
  n140 = xnode "VI-Defined FIFO Configuration"() -> ("FIFO Out"=w4:refnum<k21>)
  n141 = node-c288() -> (w11:T2)  [unwired: 1 in]
  n142 = timed-loop {
    timing: w11 -> [_]
    timing-out: [_] -> w10
    tunnel: w4 -> [w397]
    stop <- FALSE stop-if-true
    # "SPI / CS DIO"
    # "SPI / SPI"
    # "SPI"
    n143 = xnode "FPGA I/O Node"() -> ("SPI MISO"=w414)  [unwired: 1 in, 1 out]
    n144 = call "SPI Master.vi"("Count"="SPI.SPI.CNT", "Configuration"="SPI.SPI.CNFG", "Start?"="SPI.SPI.GO", "MISO"=w414, "Data Out"="SPI.SPI.DATO") -> ("Status"=w395:u8, "SCLK"=w408:bool, "MOSI"=w409:bool, "Data In"=→"SPI.SPI.DATI":u16)  [unwired: 3 in]
    "SPI.SPI.STAT" <- w395
    n145 = xnode "FPGA I/O Node"("SPI MOSI"=w409, "SPI CLK"=w408) -> ()  [unwired: 2 in, 2 out]
    n146 = call "SPI IRQ.vi"("SPI.A.IRQ.NO"="SPI.SPI.IRQ.NO", "SPI.STAT"=w395, "FIFO In"=w397) -> ()  [unwired: 9 in]
    n147 = call "Split HDC Bank1 DIO.vi"("IN 7:0"="DIO.SPI_CS3:0.OUT") -> ("OUT 3:0"=w404:fxp<+,4,4>)  [unwired: 2 out]
    n148 = call "Split HDC Bank1 DIO.vi"("IN 7:0"="DIO.SPI_CS3:0.DIR") -> ("OUT 3:0"=w403:fxp<+,4,4>)  [unwired: 2 out]
    n149 = call "DIO 4-bit.vi"("DIO0 Refnum"=refnum<k21> "SPI CS0", "DIO1 Refnum"=refnum<k21> "SPI CS1" ("DIO0 Refnum"), "DIO2 Refnum"=refnum<k21> "SPI CS2" ("DIO0 Refnum"), "DIR 3:0"=w403, "OUT 3:0"=w404, "DIO3 Refnum"=refnum<k21> "SPI CS3" ("DIO0 Refnum")) -> ("IN 3:0"=w402:fxp<+,4,4>)  [unwired: 5 in]
    n150 = call "Join HDC Bank1 DIO.vi"("IN 3:0"=w402) -> ("OUT 7:0"=→"DIO.SPI_CS3:0.IN":u8)  [unwired: 2 in]
  }
  n151 = while {
    stop <- FALSE stop-if-true
    # "Connector SPI SPI SCTL Interrupt Buffer"
    n152 = feedback #8(u8 0 ("Element")) -> (w421:u8)
    n153 = feedback #9(FALSE ("Timed Out?")) -> (w425:bool)
    n154 = case shown="False" w425 {
      tunnel: [w427 w429] -> w422
      tunnel: w421 -> [_ w429]
      frame False {
        n155 = xnode ("FIFO Method Node")("Timeout"=-1) -> ("Element"=w427:u8)  [unwired: 1 in, 2 out]
      }
      frame True {
      }
    }
    n156 = feedback-in #8(w422) -> ()
    n157 = xnode ("FIFO Method Node")("Element"=w422, "Timeout"=0) -> ("Timed Out?"=w423:bool)  [unwired: 1 in, 1 out]
    n158 = feedback-in #9(w423) -> ()
  }
  n159 = node-c288(w10) -> ()
  n160 = node-c288() -> (w13:T2)  [unwired: 1 in]
  n161 = timed-loop {
    timing: w13 -> [_]
    timing-out: [_] -> w12
    stop <- FALSE stop-if-true
    # "I2C"
    n162 = call "DIO_I2C.vi"("I2C.CNFG"="I2C.I2C.CNFG", "I2C.CNTL"="I2C.I2C.CNTL", "I2C.ADDR"="I2C.I2CADDR", "I2C.DATO"="I2C.I2C.DATO", "DIO.1/I2C.SDA"=refnum<k21> "I2C SDA" ("FPGA I/O In"), "I2C.CNTR"="I2C.I2C.CNTR", "DIO.0/I2C.SCL"=refnum<k21> "I2C SCL" ("FPGA I/O In"), "Execute?"="I2C.I2C.GO", "SELECT"=TRUE) -> ("I2C.DATI"=→"I2C.I2C.DATI":u8, "I2C.STAT"=→"I2C.I2C.STAT":u8)  [unwired: 8 in, 1 out]
  }
  n163 = node-c288(w12) -> ()
  n164 = node-c288() -> (w17:T2)  [unwired: 1 in]
  n165 = timed-loop {
    timing: w17 -> [_]
    timing-out: [_] -> w16
    stop <- FALSE stop-if-true
    # "Relay"
    n166 = Number To Boolean Array(number="DO.RELAY.OUT") -> (Boolean array=w452:bool[])
    n167 = Index Array(array=w452) -> (element #1=w451:bool, element #2=w450:bool, element #3=w449:bool, element #4=w448:bool, element #5=w447:bool, element #6=w446:bool, element #7=w445:bool, element #8=w444:bool)  [unwired: 8 in]
    n168 = xnode "FPGA I/O Node"("RelayFwd0"=w451, "RelayRev0"=w450, "RelayFwd1"=w449, "RelayRev1"=w448, "RelayFwd2"=w447, "RelayRev2"=w446, "RelayFwd3"=w445, "RelayRev3"=w444) -> ()  [unwired: 8 in, 8 out]
  }
  n169 = node-c288(w16) -> ()
  n170 = node-c288() -> (w9:T2)  [unwired: 1 in]
  n171 = timed-loop {
    timing: w9 -> [_]
    timing-out: [_] -> w8
    stop <- FALSE stop-if-true
    # "RSL"
    n172 = xnode "FPGA I/O Node"("RSL"="DO.RSL.OUT") -> ()  [unwired: 1 in, 1 out]
  }
  n173 = node-c288(w8) -> ()
